vi "For loop Tunnel.vi"() -> ()   [LabVIEW 2015]
panel:
  in  "Tab Control":enum32{"Page 1", "Page 2"}(tab)
  out "Array":i32[](array[numeric])
  # "For loop Tunnel"
  # "Pardeep Kumar"
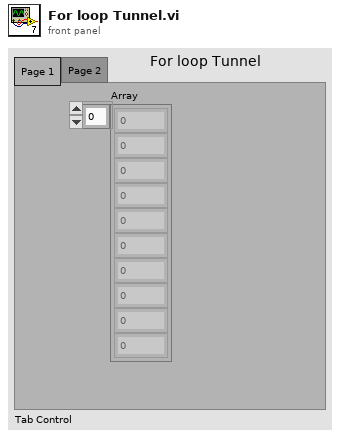
[diagram p1: front panel]
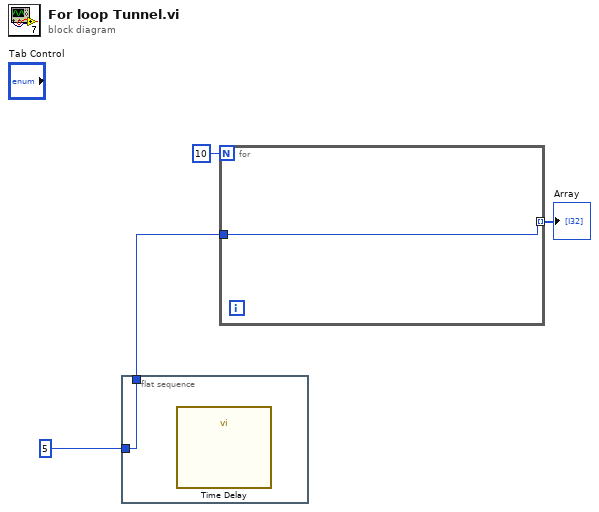
[diagram p0: block diagram]
diagram:
  n1 = flat-sequence {
    tunnel: 5 -> [w5]
    tunnel: [w5] -> w2
    frame #0 {
      n2 = call "Time Delay"() -> ()  [unwired: 11 in, 1 out]
    }
  }
  n3 = for {
    N: 10 -> [_]
    tunnel: [w6] -> w1 mode=indexing
    tunnel: w2 -> [w6]
  }
  "Array" <- w1
